vi "readConfig_DeviceInit.vi"(0 "cam calib":T7={"incident ANGLE COMPENSATION"=[], "dp/B [MeV/C/B]"=[], "charge compensation"=[], "Momentum [MeV/C]"=[], "energyDependence Input"=[], "pixel angle (y)"=[], "dp [MeV/C/] "=[], "angle 2Dfor spectrumj"=[], "dp [MeV/C] 2D"=[], "charge compensation 2D"=[], "Screen&Camera 2"={"Screen Orientation"="Regular", "Screen angle"="Flat", "Lens"=enum."FL1-f8x08", "Calibration (mm/pix)"=1.0}, "ROI info"={"npix-X"=0, "npix-Y"=0, "Left [pix]"=0.0, "Top [pix]"=0.0}, "Y 2D full angle"=[], "calib pixel"={"y1(pixel)"=[], "y2(pixel)"=[], "dp/B [MeV/C/B] (pixel)"=[], "energyDependence Input(pixel)"=[], "bending angle [deg](pixel)"=[], "total path(pixel)"=[], "pixel angle (y)(pixel)"=[], "energy dependence (pixel)"=[], "charge compensation (pixel)"=[], "Momentum [MeV/C](pixel)"=[], "angular compensation(pixel)"=[]}, "2D"={"dp"=[], "chargeCompensation"=[], "angle"=[], "Momentum"=[]}, "UserROI"={"Width"=0.0, "Hight"=0.0, "OffsetX"=0.0, "OffsetY"=0.0}, "final"={"X"=[], "xi"=[], "delta momentum"=0.0, "Y"=[], "yi"=[], "angle (Y)"=[], "delta angle"=0.0, "scale delta angle"=0.0, "intraX"=0.0, "intraY"=0.0, "mask"=[]}, "B[T]"=1.0, "index"=0.0}, 1 "B [T]":dbl=1.0, 5 "Cam 0":T1={"position"=0.0, "pixelsize"=0.0, "start"=0.0, "end"=0.0, "center"=0.0, "Lens"=enum."FL1-f8x08", "Forward"=enum."off", "Spec_Calib_file 2"=path "Y:/100TWdata/ESMCalib/datFwd.txt", "map"=path "Y:/100TWdata/ESMCalib/mapFwd.txt", "y size"=0, "UserROI"={"Width"={"Value"=0.0, "Min"=0.0, "Max"=0.0, "StepSize"=0.0, "Tolerance"=0.0, "ValueActual"=0.0}, "Hight"={"Value"=0.0, "Min"=0.0, "Max"=0.0, "StepSize"=0.0, "Tolerance"=0.0, "ValueActual"=0.0}, "OffsetX"={"Value"=0.0, "Min"=0.0, "Max"=0.0, "StepSize"=0.0, "Tolerance"=0.0, "ValueActual"=0.0}, "OffsetY"={"Value"=0.0, "Min"=0.0, "Max"=0.0, "StepSize"=0.0, "Tolerance"=0.0, "ValueActual"=0.0}}, "CamMaxPixel"={"X"=0, "Y"=0}, "CamROI"={"Width"=0.0, "Hight"=0.0, "OffsetX"=0.0, "OffsetY"=0.0}}, 11 "error in (no error)":errorcluster) -> (4 "Cam calib":T7={"incident ANGLE COMPENSATION"=[], "dp/B [MeV/C/B]"=[], "charge compensation"=[], "Momentum [MeV/C]"=[], "energyDependence Input"=[], "pixel angle (y)"=[], "dp [MeV/C/] "=[], "angle 2Dfor spectrumj"=[], "dp [MeV/C] 2D"=[], "charge compensation 2D"=[], "Screen&Camera 2"={"Screen Orientation"="Regular", "Screen angle"="Flat", "Lens"=enum."FL1-f8x08", "Calibration (mm/pix)"=1.0}, "ROI info"={"npix-X"=0, "npix-Y"=0, "Left [pix]"=0.0, "Top [pix]"=0.0}, "Y 2D full angle"=[], "calib pixel"={"y1(pixel)"=[], "y2(pixel)"=[], "dp/B [MeV/C/B] (pixel)"=[], "energyDependence Input(pixel)"=[], "bending angle [deg](pixel)"=[], "total path(pixel)"=[], "pixel angle (y)(pixel)"=[], "energy dependence (pixel)"=[], "charge compensation (pixel)"=[], "Momentum [MeV/C](pixel)"=[], "angular compensation(pixel)"=[]}, "2D"={"dp"=[], "chargeCompensation"=[], "angle"=[], "Momentum"=[]}, "UserROI"={"Width"=0.0, "Hight"=0.0, "OffsetX"=0.0, "OffsetY"=0.0}, "final"={"X"=[], "xi"=[], "delta momentum"=0.0, "Y"=[], "yi"=[], "angle (Y)"=[], "delta angle"=0.0, "scale delta angle"=0.0, "intraX"=0.0, "intraY"=0.0, "mask"=[]}, "B[T]"=1.0, "index"=0.0}, 15 "error out":errorcluster)   [LabVIEW 2020]
uses:
  calib_Sub_Typdef.ctl
  OnOffTypeDef.ctl
  CamSettingSUB_TypDEf.ctl
  ROIInfo_TypDef.ctl
  CamAndObj_TypDEf.ctl
  ScreenCam2_TypDEf.ctl
  source/Device Drivers/shared/numericVariable_TypeDef.ctl
  source/Device Drivers/BaseDriver/BaseDriver.lvclass
  userROI.ctl
  CamRoiTypDef.ctl
  calibPixel.ctl
  2DTypDef.ctl
  finalCalibTypdef.ctl
panel:
  out "XY Graph":cluster{dbl[], "Array out":dbl[]}[](graph)
  out "angular compensation(pixel)":dbl[](graph)=[0.8828668755883531, 0.8822731719380749, 0.8816794682877969, 0.8810857646375188, 0.8804920609872405, 0.8798983573369628, 0.8793046536866845, 0.8786938174428058, 0.878070999398585, 0.8774481813543642, 0.8768253633101438, 0.8762025452659231, 0.8755797272217022, 0.8749569091774815, 0.8743340911332609, 0.8737112730890402, 0.8730884550448196, 0.8724656370005986, 0.871842818956378, 0.8712200009121572, 0.8705971828679367, 0.869974364823716, 0.8693515467794952, 0.8687287287352744, 0.8681059106910538, 0.8674830926468331, 0.8668602746026125, 0.8662374565583917, 0.865614638514171, 0.8649839877329895, 0.8643469373942262, 0.8637098870554627, 0.8630728367166994, 0.8624357863779362, 0.8617987360391728, 0.8611616857004095, 0.8605246353616463, 0.859887585022883, 0.8592505346841194, 0.8586134843453561, 0.8579764340065928, 0.8573393836678295, 0.8567023333290662, 0.8560652829903028, 0.8554282326515393, 0.8547911823127761, 0.8541541319740128, 0.8535170816352496, 0.852880031296486, 0.8522429809577228, 0.8516082170315974, 0.850974837169528, 0.8503414573074587, 0.8497080774453892, 0.8490746975833201, 0.8484413177212509, 0.8478079378591814, 0.847174557997112, 0.8465411781350429, 0.8459077982729736, 0.8452744184109042, 0.844641038548835, 0.8440076586867656, 0.8433742788246964, 0.8427408989626272, 0.8421075191005577, 0.8414741392384882, 0.840840759376419, 0.8402073795143499, 0.8395739996522804, 0.8389344428970866, 0.838264939549894, 0.8375954362027014, 0.8369259328555086, 0.8362564295083159, 0.8355869261611232, 0.8349174228139307, 0.8342479194667378, 0.8335784161195451, 0.8329089127723526, 0.8322394094251598, 0.831569906077967, 0.8309004027307744, 0.8302308993835817, 0.829561396036389, 0.8288918926891963, 0.8282223893420035, 0.8275528859948109, 0.8268833826476183, 0.8262071159329748, 0.8255192546584292, 0.824831393383884, 0.8241435321093383, 0.823455670834793, 0.8227678095602475, 0.822079948285702, 0.8213920870111564, 0.8207042257366111, 0.8200163644620655, 0.8193285031875202, 0.8186406419129747, 0.817952780638429, 0.8172649193638838, 0.8165770580893382, 0.8158891968147929, 0.8152013355402473, 0.8145134742657018, 0.8138275052588367, 0.8131429262966198, 0.8124583473344027, 0.8117737683721855, 0.8110891894099685, 0.8104046104477516, 0.8097200314855346, 0.8090354525233175, 0.8083508735611004, 0.8076662945988833, 0.8069817156366664, 0.8062971366744494, 0.8056125577122323, 0.804927978750015, 0.8042433997877982, 0.803558820825581, 0.8028742418633639, 0.802185846968365, 0.8014809873492605, 0.8007761277301558, 0.8000712681110512, 0.7993664084919465, 0.7986615488728418, 0.7979566892537374, 0.7972518296346326, 0.7965469700155281, 0.7958421103964233, 0.7951372507773187, 0.794432391158214, 0.7937275315391092, 0.7930226719200049, 0.7923178123009001, 0.7916129526817955, 0.7909080930626908, 0.7902056488450743, 0.7895039617779784, 0.7888022747108826, 0.7881005876437865, 0.7873989005766904, 0.7866972135095943, 0.7859955264424984, 0.7852938393754024, 0.7845921523083065, 0.7838904652412104, 0.7831887781741143, 0.7824870911070184, 0.7817854040399225, 0.7810837169728263, 0.7803820299057302, 0.7796803428386344, 0.7789542032331801, 0.7782178197397002, 0.7774814362462202, 0.7767450527527405, 0.7760086692592606, 0.7752722857657809, 0.774535902272301, 0.7737995187788212, 0.7730631352853413, 0.7723267517918616, 0.7715903682983818, 0.7708539848049022, 0.7701176013114223, 0.7693812178179424, 0.7686448343244626, 0.7679084508309829, 0.767172067337503, 0.7664356838440229, 0.7656993003505433, 0.7649629168570634, 0.7642265333635837, 0.7634901498701038, 0.7627537663766243, 0.7620173828831442, 0.7612809993896646, 0.7605446158961846, 0.759808232402705, 0.759071848909225, 0.7583354654157451, 0.7575918748584242, 0.7568323364584342, 0.7560727980584444, 0.7553132596584544, 0.7545537212584644, 0.7537941828584744, 0.7530346444584847, 0.7522751060584949, 0.7515155676585048, 0.7507560292585148, 0.749996490858525, 0.7492369524585353, 0.7484774140585454, 0.7477178756585553, 0.7469583372585653, 0.7461987988585754, 0.7454392604585857, 0.7446797220585957, 0.7439201836586059, 0.7431606452586157, 0.7424011068586259, 0.7416415684586358, 0.7408820300586461, 0.740122491658656, 0.7393629532586662, 0.7386034148586762, 0.7378438764586863, 0.737081451735524, 0.7363116502591329, 0.735541848782742, 0.7347720473063514, 0.7340022458299608, 0.7332324443535698, 0.7324626428771788, 0.7316928414007882, 0.7309230399243972, 0.7301532384480066, 0.7293834369716157, 0.7286136354952251, 0.727843834018834, 0.7270740325424433, 0.7263042310660524, 0.7255344295896617, 0.7247646281132708, 0.7239948266368798, 0.7232250251604891, 0.7224552236840982, 0.7216854222077076, 0.7209156207313165, 0.7201458192549259, 0.719376017778535, 0.7186062163021444, 0.7178364148257533, 0.717039349891366, 0.7162408936596031, 0.7154424374278405, 0.7146439811960779, 0.7138455249643151, 0.7130470687325524, 0.7122486125007894, 0.7114501562690269, 0.7106517000372643, 0.7098532438055013, 0.7090547875737387, 0.708256331341976, 0.7074578751102132, 0.7066594188784505, 0.7058609626466877, 0.7050625064149252, 0.7042640501831622, 0.7034655939513996, 0.702667137719637, 0.701868681487874, 0.7010702252561114, 0.7002717690243486, 0.6994733127925858, 0.6986648856562896, 0.6978529139188272, 0.6970409421813651, 0.6962289704439028, 0.6954169987064405, 0.694605026968978, 0.6937930552315159, 0.6929810834940539, 0.6921691117565915, 0.6913571400191291, 0.6905451682816669, 0.6897331965442048, 0.6889212248067424, 0.6881092530692801, 0.6872972813318179, 0.6864853095943557, 0.6856733378568937, 0.6848613661194313, 0.6840493943819689, 0.6832374226445068, 0.6824254509070444, 0.6816130566207561, 0.680765735185049, 0.6799184137493418, 0.6790710923136346, 0.6782237708779276, 0.6773764494422206, 0.6765291280065137, 0.6756818065708063, 0.6748344851350991, 0.6739871636993923, 0.6731398422636852, 0.6722925208279781, 0.671445199392271, 0.670597877956564, 0.6697505565208568, 0.6689032350851498, 0.6680559136494427, 0.6672085922137355, 0.6663612707780286, 0.6655139493423214, 0.6646674205061246, 0.663824474080577, 0.6629815276550295, 0.6621385812294818, 0.6612956348039342, 0.6604526883783869, 0.6596097419528393, 0.6587667955272917, 0.6579238491017441, 0.6570809026761967, 0.6562379562506491, 0.6553950098251016, 0.6545520633995541, 0.6537091169740062, 0.652866170548459, 0.6520232241229114, 0.6511802776973638, 0.650337331271816, 0.6494943848462685, 0.6486483354760286, 0.6477871135930843, 0.6469258917101401, 0.6460646698271957, 0.6452034479442517, 0.6443422260613073, 0.643481004178363, 0.6426197822954187, 0.6417585604124744, 0.6408973385295303, 0.640036116646586, 0.6391748947636416, 0.6383136728806974, 0.6374524509977529, 0.6365912291148087, 0.6357300072318647, 0.6348687853489202, 0.634007563465976, 0.6331279837920514, 0.6322217346462464, 0.6313154855004414, 0.6304092363546362, 0.6295029872088311, 0.6285967380630261, 0.6276904889172212, 0.6267842397714162, 0.6258779906256108, 0.6249717414798057, 0.6240654923340009, 0.6231592431881958, 0.6222529940423908, 0.6213467448965855, 0.6204404957507805, 0.6195342466049755, 0.6186362319196459, 0.6177591120479985, 0.6168819921763513, 0.6160048723047041, 0.6151277524330566, 0.6142506325614094, 0.6133735126897623, 0.6124963928181149, 0.6116192729464677, 0.6107421530748205, 0.6098650332031732, 0.6089879133315259, 0.6081107934598786, 0.6072336735882314, 0.606356553716584, 0.6054794338449367, 0.6045849033396737, 0.6036576331986484, 0.6027303630576228, 0.6018030929165974, 0.6008758227755718, 0.5999485526345464, 0.5990212824935209, 0.5980940123524955, 0.59716674221147, 0.5962394720704444, 0.595312201929419, 0.5943849317883936, 0.5934576616473679, 0.5925303915063426, 0.5916031213653172, 0.5906788745779357, 0.5897548821929486, 0.5888308898079617, 0.5879068974229748, 0.586982905037988, 0.586058912653001, 0.5851349202680142, 0.584210927883027, 0.5832869354980402, 0.5823629431130533, 0.5814389507280664, 0.5805149583430794, 0.5795909659580926, 0.5786655044856217, 0.5777142146141486, 0.5767629247426757, 0.5758116348712025, 0.5748603449997295, 0.5739090551282565, 0.5729577652567832, 0.5720064753853101, 0.5710551855138369, 0.5701038956423641, 0.569152605770891, 0.5682013158994178, 0.5672500260279447, 0.5662991447514474, 0.5653507782816504, 0.5644024118118531, 0.563454045342056, 0.562505678872259, 0.5615573124024618, 0.5606089459326647, 0.5596605794628674, 0.5587122129930703, 0.5577638465232732, 0.556815480053476, 0.5558671135836789, 0.5549187471138817, 0.5539721633480208, 0.553026307753077, 0.5520804521581331, 0.5511345965631893, 0.5501887409682453, 0.5492428853733015, 0.5482970297783576, 0.5473511741834136, 0.5464053185884699, 0.5454594629935259, 0.544513607398582, 0.5435677518036383, 0.5425986950895735, 0.5416215579058994, 0.5406444207222251, 0.5396672835385506, 0.5386901463548764, 0.5377130091712021, 0.5367358719875279, 0.5357587348038535, 0.5347815976201793, 0.5338044604365049, 0.5328273232528304, 0.5318516616677071, 0.5308769421669517, 0.5299022226661962, 0.5289275031654408, 0.5279527836646853, 0.5269780641639299, 0.5260033446631744, 0.525028625162419, 0.5240539056616635, 0.5230791861609082, 0.5221044666601528, 0.521131666614299, 0.5201591306932939, 0.5191865947722889, 0.5182140588512839, 0.517241522930279, 0.5162689870092739, 0.5152964510882689, 0.514323915167264, 0.5133513792462588, 0.512378843325254, 0.5113871877086447, 0.5103784744313514, 0.5093697611540582, 0.5083610478767651, 0.5073523345994718, 0.5063436213221787, 0.5053349080448855, 0.5043261947675923, 0.5033174814902991, 0.5023087682130059, 0.5013018429816303, 0.5002950728850671, 0.49928830278850395, 0.4982815326919408, 0.4972747625953776, 0.49626799249881454, 0.4952612224022513, 0.4942544523056882, 0.49324768220912496, 0.4922292975600831, 0.4912044771524138, 0.49017965674474434, 0.48915483633707496, 0.4881300159294059, 0.48710519552173653, 0.48608037511406715, 0.4850555547063979, 0.4840307342987285, 0.48300591389105907, 0.48198109348338997, 0.4809562730757207, 0.47993145266805126, 0.47890663226038194, 0.47788181185271256, 0.47685699144504345, 0.4758321710373741, 0.47480010738587114, 0.4737562099821137, 0.47271231257835633, 0.4716684151745989, 0.4706245177708415, 0.4695806203670842]
  out "Momentum [MeV/C](pixel)":dbl[](graph)
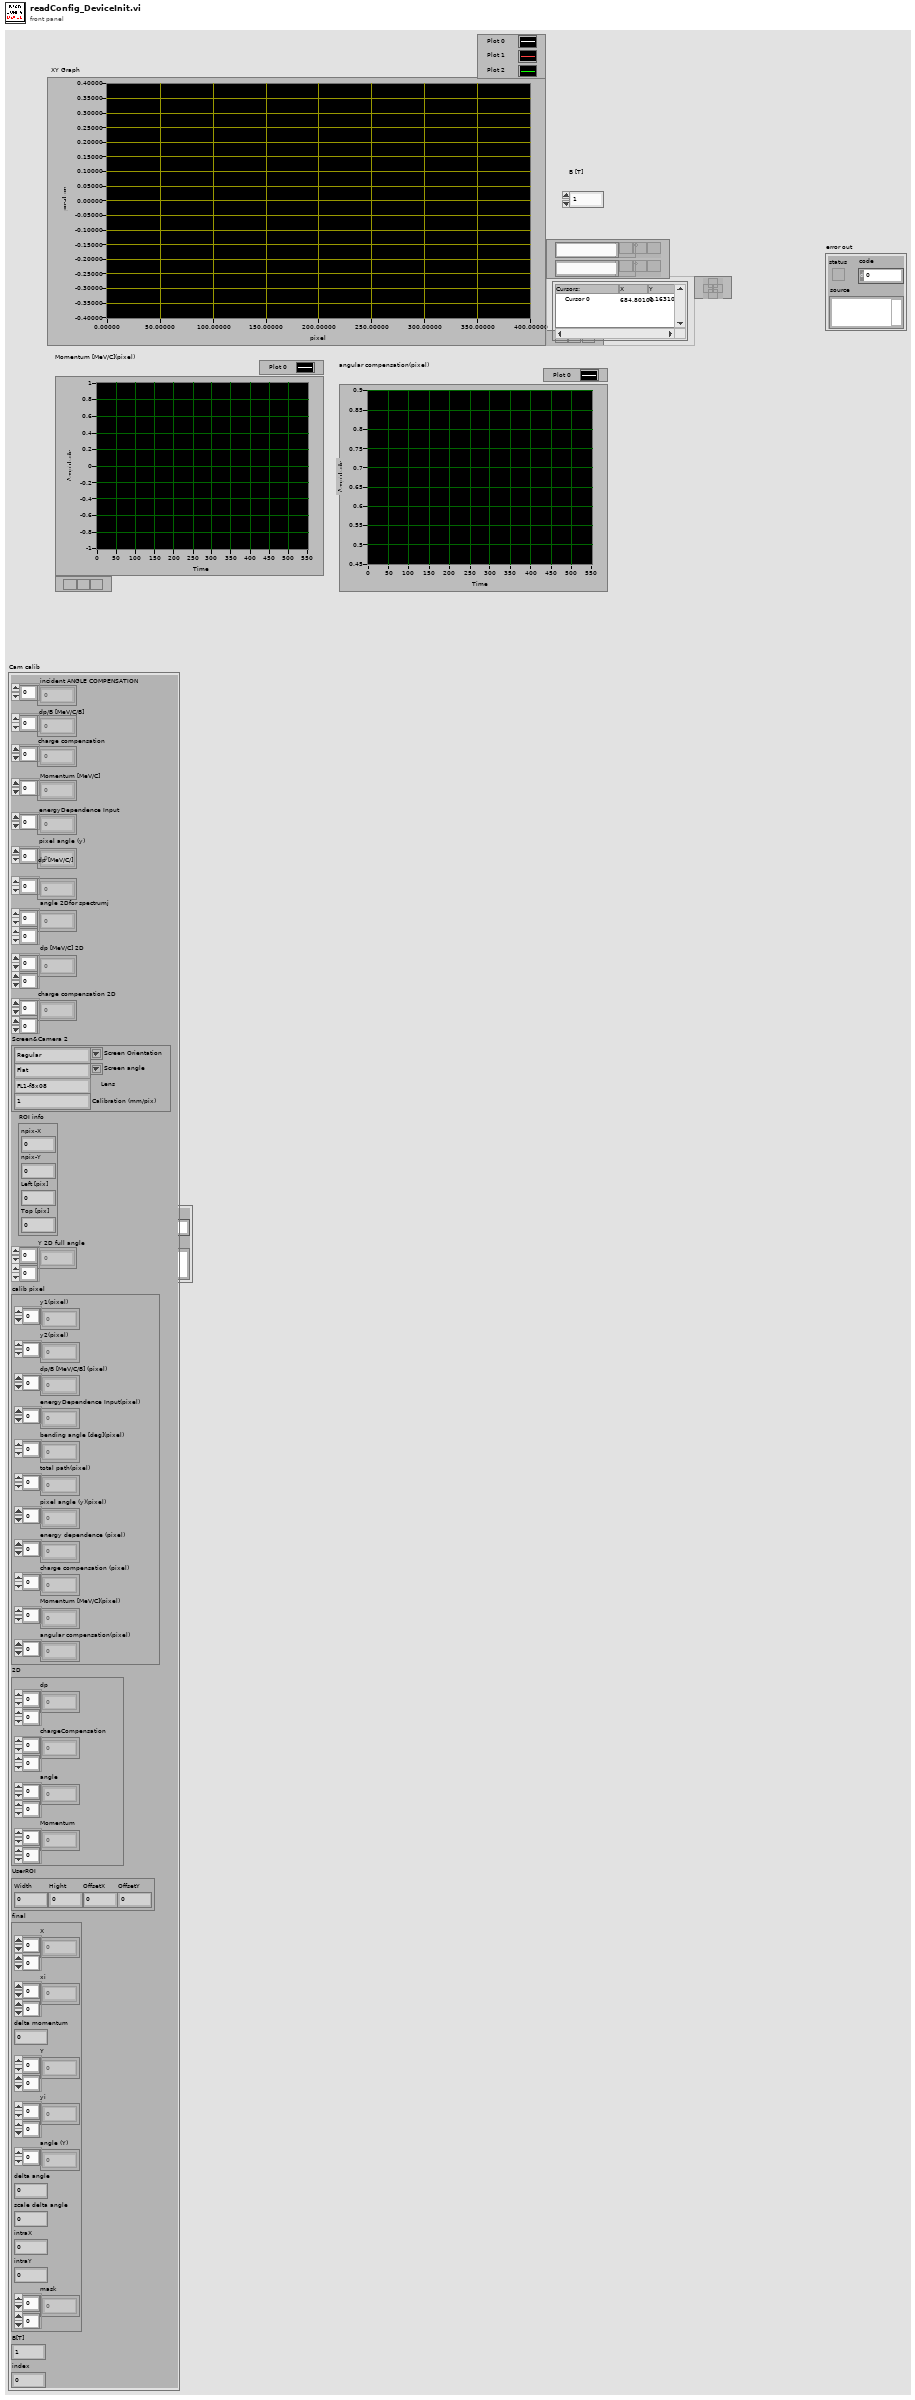
[diagram p1: front panel]
types:
  T1 = typedef "CamSettingSUB_TypDEf.ctl" = cluster{"position":dbl, "pixelsize":dbl, "start":dbl, "end":dbl, "center":dbl, "Lens":T2, "Forward":T3, "Spec_Calib_file 2":path, "map":path, "y size":i32, "UserROI":T4, "CamMaxPixel":cluster{"X":i32, "Y":i32}, "CamROI":T6}
  T2 = typedef "CamAndObj_TypDEf.ctl" = enum16{"FL1-f8x08", "FL1-f8x06", "FL1-f8", "ch300-f50", "FL2G-f8", "FL3M14-f8", "FL3M14-f8x08", "FL3M14-f8x08(2x2)"}
  T3 = typedef "OnOffTypeDef.ctl" = enum16{"off", "on"}
  T4 = typedef "userROI.ctl" = cluster{"Width":T5, "Hight":T5, "OffsetX":T5, "OffsetY":T5}
  T5 = typedef "BaseDriver.lvclass/numericVariable_TypeDef.ctl" = cluster{"Value":dbl, "Min":dbl, "Max":dbl, "StepSize":dbl, "Tolerance":dbl, "ValueActual":dbl}
  T6 = typedef "CamRoiTypDef.ctl" = cluster{"Width":dbl, "Hight":dbl, "OffsetX":dbl, "OffsetY":dbl}
  T7 = typedef "calib_Sub_Typdef.ctl" = cluster{"incident ANGLE COMPENSATION":dbl[], "dp/B [MeV/C/B]":dbl[], "charge compensation":dbl[], "Momentum [MeV/C]":dbl[], "energyDependence Input":dbl[], "pixel angle (y)":dbl[], "dp [MeV/C/] ":dbl[], "angle 2Dfor spectrumj":dbl[][], "dp [MeV/C] 2D":dbl[][], "charge compensation 2D":dbl[][], "Screen&Camera 2":T8, "ROI info":T9, "Y 2D full angle":dbl[][], "calib pixel":T10, "2D":T11, "UserROI":T6, "final":T12, "B[T]":dbl, "index":dbl}
  T8 = typedef "ScreenCam2_TypDEf.ctl" = cluster{"Screen Orientation":string, "Screen angle":string, "Lens":T2, "Calibration (mm/pix)":dbl}
  T9 = typedef "ROIInfo_TypDef.ctl" = cluster{"npix-X":i32, "npix-Y":i32, "Left [pix]":dbl, "Top [pix]":dbl}
  T10 = typedef "calibPixel.ctl" = cluster{"y1(pixel)":dbl[], "y2(pixel)":dbl[], "dp/B [MeV/C/B] (pixel)":dbl[], "energyDependence Input(pixel)":dbl[], "bending angle [deg](pixel)":dbl[], "total path(pixel)":dbl[], "pixel angle (y)(pixel)":dbl[], "energy dependence (pixel)":dbl[], "charge compensation (pixel)":dbl[], "Momentum [MeV/C](pixel)":dbl[], "angular compensation(pixel)":dbl[]}
  T11 = typedef "2DTypDef.ctl" = cluster{"dp":dbl[][], "chargeCompensation":dbl[][], "angle":dbl[][], "Momentum":dbl[][]}
  T12 = typedef "finalCalibTypdef.ctl" = cluster{"X":dbl[][], "xi":dbl[][], "delta momentum":dbl, "Y":dbl[][], "yi":dbl[][], "angle (Y)":dbl[], "delta angle":dbl, "scale delta angle":dbl, "intraX":dbl, "intraY":dbl, "mask":dbl[][]}
  T13 = typedef "configTypDEf.ctl" = cluster{"bending angle":dbl[], "screen [m]":dbl[], "momentum [MeV/c]":dbl[], "total path [m]":dbl[], "x[mm](rms)":dbl[], "x[mm](rms,b)":dbl[], "y[mm](rms)":dbl[], "y[mm](rms,b)":dbl[]}
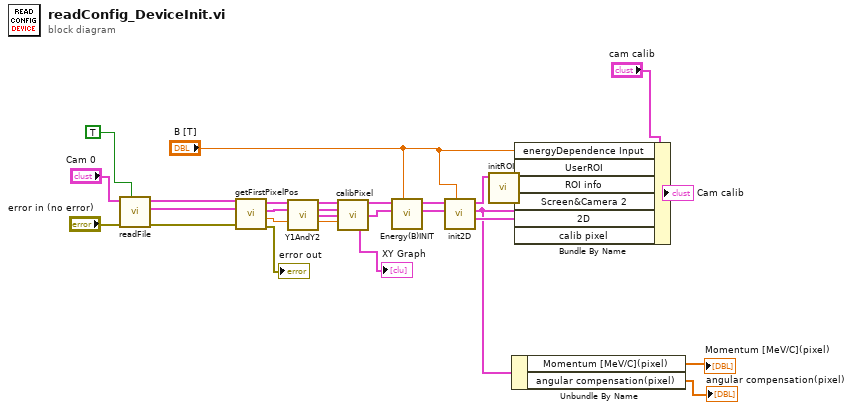
[diagram p0: block diagram]
diagram:
  n1 = call "readFile.vi"("New (one file)"=TRUE, "error in (no error)"="error in (no error)", "Cam 1"="Cam 0") -> ("error out"=w23:errorcluster, "Cluster"=w24:T13, "Cam 0"=w10:T1)  [unwired: 6 in]
  n2 = call "getFirstPixelPos.vi"("error in (no error)"=w23, "Cluster"=w24, "Cam 0"=w10) -> ("error out"=→"error out":errorcluster, "first Pixel position"=w21:dbl, "Cluster out"=w25:T13, "Cam out"=w9:T1)  [unwired: 5 in]
  n3 = call "Y1AndY2.vi"("Cam 0"=w9, "Cluster"=w25, "position"=w21) -> ("Cam 1"=w8:T1, "Clustero ut"=w20:T13, "calib(pixel)"=w19:T10, "position 2"=w18:dbl)  [unwired: 9 in]
  n4 = call "calibPixel.vi"("Cam 1"=w8, "Clustero ut"=w20, "calib(pixel) in"=w19, "first Pixel position"=w18) -> ("Cam out"=w7:T1, "calib(pixel) out"=w14:T10, "XY Graph"=→"XY Graph":cluster{dbl[], "Array out":dbl[]}[])  [unwired: 9 in]
  n5 = call "Energy(B)INIT.vi"("B [T] in"="B [T]", "calib(pixel) out in"=w14, "Cam in"=w7) -> ("calib(pixel) out out"=w13:T10, "Cam out 2"=w6:T1)  [unwired: 7 in]
  n6 = call "init2D.vi"("B [T]"="B [T]", "calib(pixel) out out"=w13, "Cam out"=w6) -> ("2D"=w12:T11, "calib(pixel) out out 2"=w3:T10, "Cam out 2"=w5:T1)  [unwired: 6 in]
  n7 = call "initROI.vi"("Cam out"=w5) -> ("Screen&Camera 2"=w16:T8, "ROI info"=w28:T9, "UserROI"=w15:T6)  [unwired: 8 in]
  n8 = Unbundle By Name(w3) -> ("Momentum [MeV/C](pixel)"=→"Momentum [MeV/C](pixel)":dbl[], "angular compensation(pixel)"=→"angular compensation(pixel)":dbl[])
  n9 = Bundle By Name(cluster="cam calib", "energyDependence Input"="B [T]", "UserROI"=w15, "ROI info"=w28, "Screen&Camera 2"=w16, "2D"=w12, "calib pixel"=w3) -> (→"Cam calib":T7)
